vi "Test.vi"(11 "ActionStack String":string="James >> T\nAnd >> F\nLucy >> i32: 64\nHave >> d: 1.12 //Comment\nFun >> 1000\n") -> (3 "Payloads":variant[](array[variant]), 5 "Actions":string[](array[string]))   [LabVIEW 2025]
uses:
  Action.lvclass/Action.ctl
panel:
  in  "path arg":path=path "C:/Program Files"
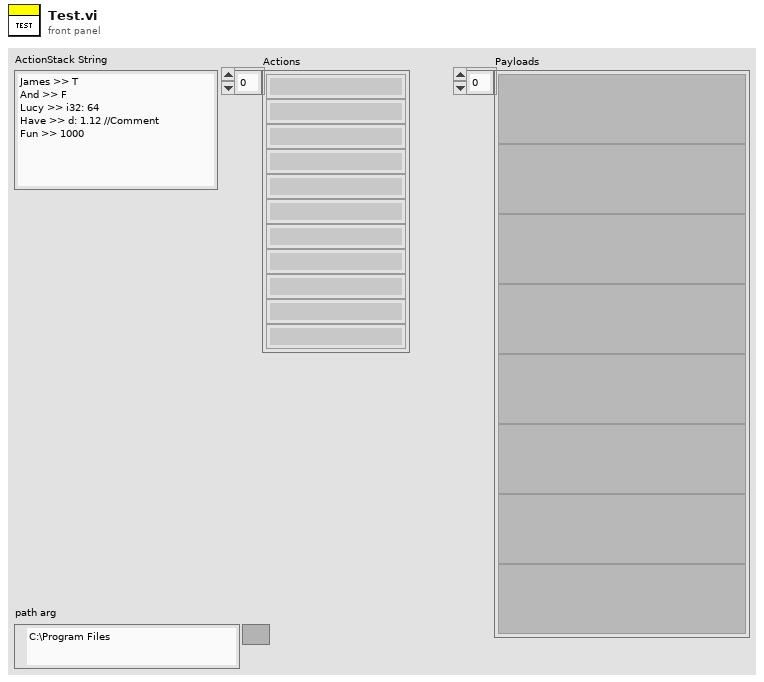
[diagram p1: front panel]
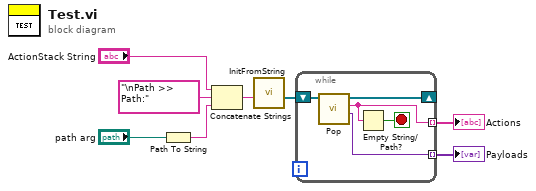
[diagram p0: block diagram]
diagram:
  n1 = Path To String(path="path arg") -> (string=w3:string)
  n2 = Concatenate Strings("ActionStack String", "\nPath >> Path:" ("string"), w3) -> (w2:string)
  n3 = call "InitFromString.vi"("ActionStack String"=w2) -> ("ActionStack out"=w1:refnum<class "Action.lvclass">[])  [unwired: 10 in]
  n4 = while {
    shift-right: [w12] -> _
    shift-left: w1 -> [w13]
    tunnel: [w11] -> w8 mode=indexing
    tunnel: [w9] -> w4 mode=indexing
    stop <- w10 stop-if-true
    n5 = call "Pop.vi"("ActionStack in"=w13) -> ("Popped Payload"=w9:variant, "Popped Action"=w11:string, "Future ActionStack"=w12:refnum<class "Action.lvclass">[])  [unwired: 8 in]
    n6 = Empty String/Path?(string/path=w11) -> (empty?=w10:bool)
  }
  "Actions" <- w8
  "Payloads" <- w4
